vi "ReceiveChatMsg.vi"(8 "error in (no error)":errorcluster, 10 "ChatMsg":string, 11 "Server in":refnum<class "Server.lvclass">) -> (0 "error out":errorcluster, 3 "Server out":refnum<class "Server.lvclass">)   [LabVIEW 2021, in "Server.lvlib" / "Server.lvclass"]
uses:
  Server.lvclass
  Server.lvclass/Server.ctl
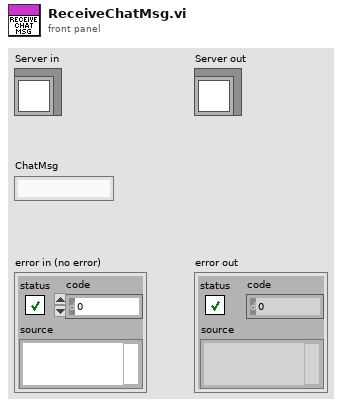
[diagram p1: front panel]
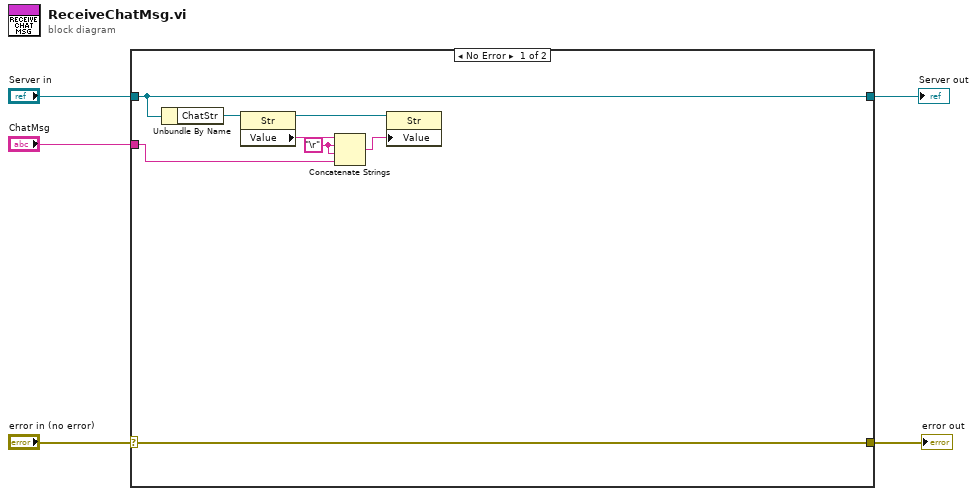
[diagram p0: block diagram]
diagram:
  n1 = case shown="No Error" "error in (no error)" {
    selector: "error in (no error)" -> [w13 w14]
    tunnel: [w13 w14] -> w1
    tunnel: "Server in" -> [w12 w15]
    tunnel: [w12 w15] -> w2
    tunnel: "ChatMsg" -> [w6 _]
    frame No Error {
      w9 = "\r"
      n2 = Unbundle By Name(w12) -> ("ChatStr"=w11:refnum<vi>)
      n3 = property class="Str"(reference=w11) -> (reference out=w8:refnum<vi>, "Value"=w10:string)  [unwired: 1 in, 1 out]
      n4 = Concatenate Strings(w10, w9, w9, w6) -> (w7:string)
      n5 = property class="Str"(reference=w8, "Value"=w7) -> ()  [unwired: 1 in, 2 out]
    }
    frame Error {
    }
  }
  "error out" <- w1
  "Server out" <- w2
